vi "ErrorHandling.Gui.vi"(6 "~Shutdown visible (T)":bool=TRUE, 8 "error in (no error)":errorcluster, 10 "~ErrData":T1, 11 "~Show? (T)":bool=TRUE) -> (0 "error out":errorcluster, 2 "~shutdown?":bool)   [LabVIEW 2016]
uses:
  CitTemplate/citTemplate.errData.ctl
  EventLog/EventLog.EventSource.ctl
  ErrorHandling.Gui.Action.ctl
panel:
  out "_loop":i32(ring)=4
  in  "DetailsButton":bool
  out "~ErrorMessage":string
  in  "OKButton":bool
  in  "ShutdownButton":bool
  out "~ErrorSource":string caption="Source"
  out "~ErrorCode":i32 caption="Code"
  out "~ErrorTime":string caption="Time"
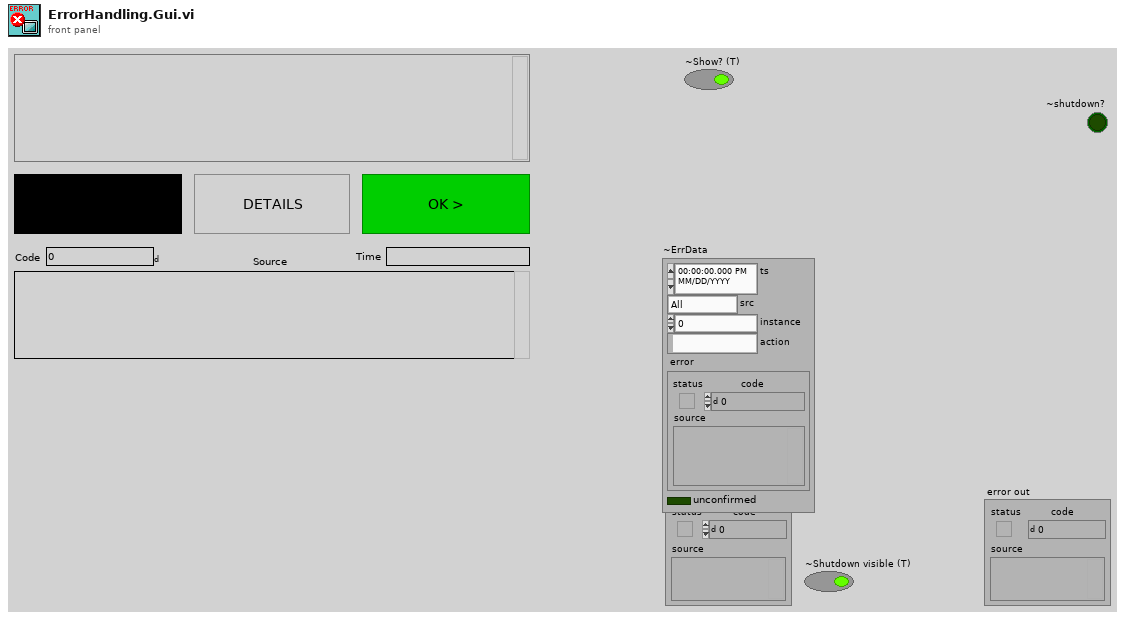
[diagram p1: front panel]
types:
  T1 = typedef "citTemplate.errData.ctl" = cluster{"ts":timestamp, "src":T2, "instance":i32, "action":string, "error":errorcluster, "unconfirmed":bool}
  T2 = typedef "EventLog.EventSource.ctl" = enum16{"All", "Gui", "Cache", "PLC1", "PLC2", "PLC3", "DB", "DB01", "DB02", "DB03", "DB04", "DB05", "DB06", "DB07", "DB08", "DB09", "DB10", "DB11", "DB12", "DB13", "DB14", "DB15", "DB16"}
  T3 = typedef "ErrorHandling.Gui.Action.ctl" = enum32{"idle", "constructor", "destructor", "--- ErrorGUI ---"}
  T4 = enum32{"invalid app kind", "Development System", "Run Time System", "Student Edition", "Embedded LabVIEW", "Evaluation", "Custom"}
  T5 = enum32{"Invalid", "Standard", "Closed", "Hidden", "Minimized", "Maximized"}
  T6 = typedef "LVRectTypeDef.ctl" = cluster{"Left":i16, "Top":i16, "Right":i16, "Bottom":i16}
  T7 = typedef "LVPositionTypeDef.ctl" = cluster{"Left":i32, "Top":i32}
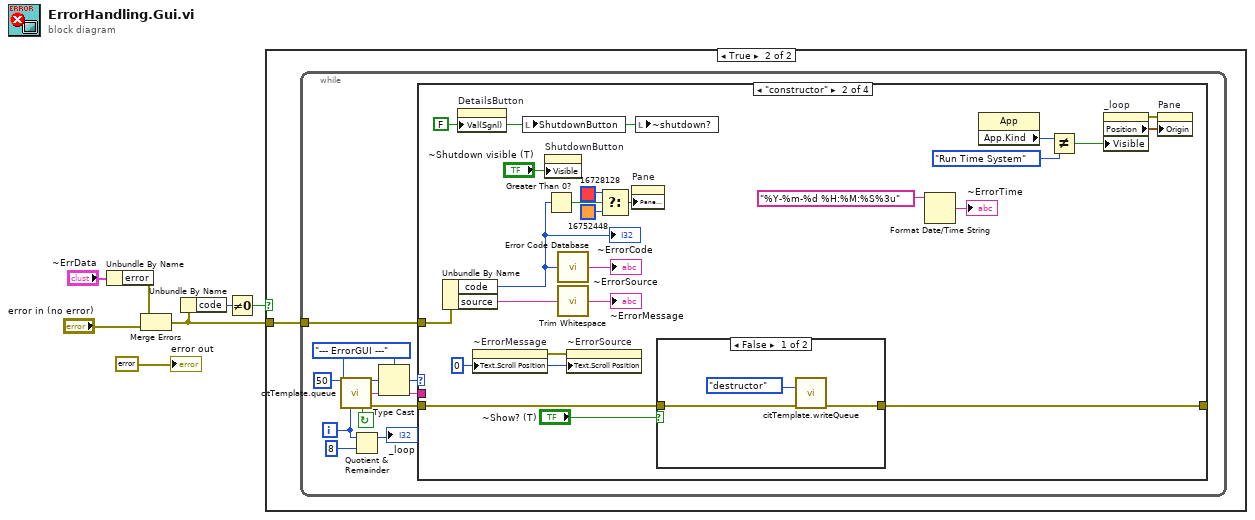
[diagram p0: block diagram]
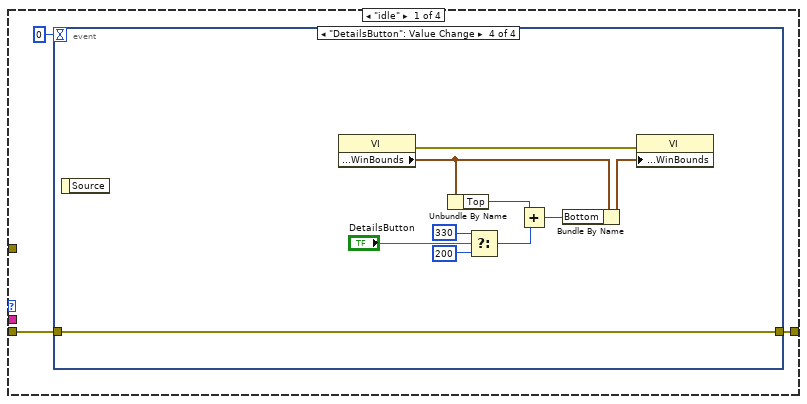
[diagram p3: hidden frame]
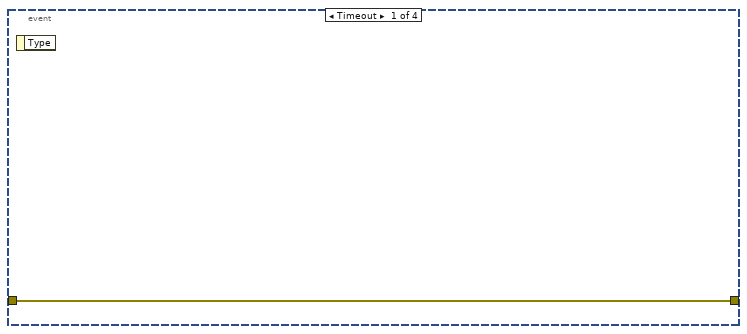
[diagram p4: hidden frame]
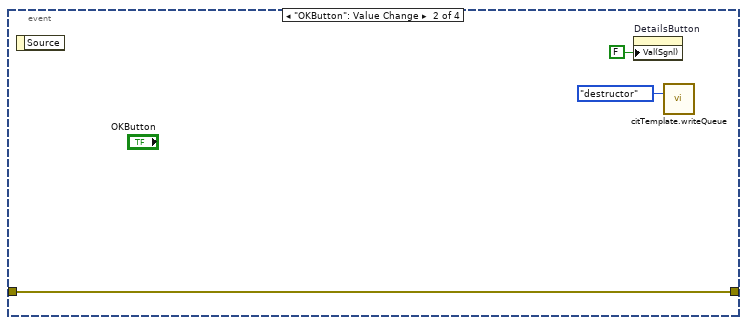
[diagram p5: hidden frame]
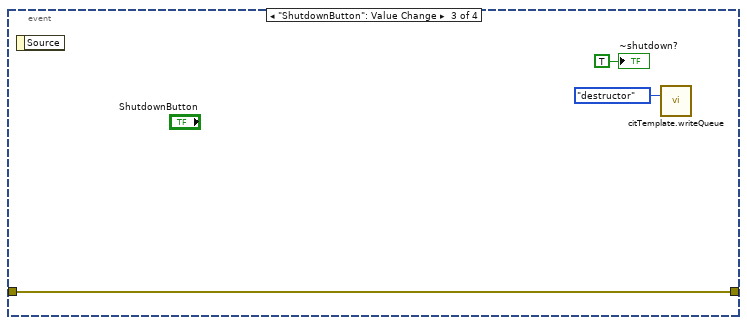
[diagram p6: hidden frame]
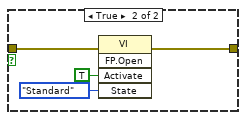
[diagram p7: hidden frame]
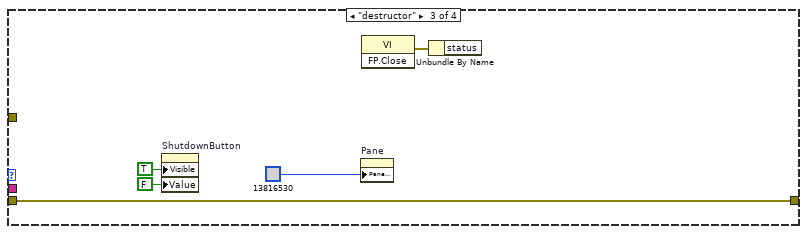
[diagram p8: hidden frame]
diagram:
  n1 = Unbundle By Name("~ErrData") -> ("error"=w2:errorcluster)
  n2 = Merge Errors(w2, "error in (no error)") -> (w3:errorcluster)
  n3 = Unbundle By Name(w3) -> ("code"=w4:i32)
  n4 = Not Equal To 0?(x=w4) -> (x != 0?=w1:bool)
  n5 = case shown="True" w1 {
    tunnel: w3 -> [_ w8]
    frame False {
    }
    frame True {
      n6 = while {
        tunnel: w8 -> [w9]
        i -> [w11]
        stop <- w19 continue-if-true
        w13 = ErrorHandling.Gui.Action."--- ErrorGUI ---" ("Action")
        n7 = call "citTemplate.queue.vi"("ms timeout (250 ms)"=50, "event enum"=w13, "iteration (-1)"=w11) -> ("event out"=w17:u32, "(flatten) data out"=w14:string, "continue"=w19:bool, "error out"=w15:errorcluster)  [unwired: 2 in, 7 out]
        n8 = Quotient & Remainder(x=w11, y=8) -> (x-y*floor(x/y)=→"_loop":i32)  [unwired: 1 out]
        n9 = Type Cast(type=w13, x=w17) -> (*(type *) &x=w16:T3)
        n10 = case shown="\"constructor\"" w16 {
          tunnel: [w20 w40 w74 w75] -> _
          tunnel: w15 -> [w21 w41 w74 w75]
          tunnel: w14 -> [_ _ _ _]
          tunnel: w9 -> [_ w53 _ _]
          frame "idle" {
            n11 = event shown="[3] \"DetailsButton\": Value Change" {
              selector: _ -> [_ _ _ _]
              dyn-events: _ -> [_ _ _ _]
              timeout: 0 -> [_ _ _ _]
              tunnel: w21 -> [w23 w25 w29 w30]
              tunnel: [w23 w25 w29 w30] -> w20
              event Timeout {
                n12 = event-data() -> ()  [unwired: 2 out]
              }
              event "OKButton": Value Change {
                n13 = event-data() -> ()  [unwired: 2 out]
                n14 = property on="DetailsButton" class="Bool (strict)"("Val(Sgnl)"=FALSE ("Value (Signaling)")) -> ()  [unwired: 2 in, 2 out]
                n15 = call "citTemplate.writeQueue.vi"("event in (if not connected:all statemachine with data event)"=ErrorHandling.Gui.Action."destructor" ("Action")) -> ()  [unwired: 4 in, 11 out]
              }
              event "ShutdownButton": Value Change {
                n16 = event-data() -> ()  [unwired: 2 out]
                n17 = call "citTemplate.writeQueue.vi"("event in (if not connected:all statemachine with data event)"=ErrorHandling.Gui.Action."destructor" ("Action")) -> ()  [unwired: 4 in, 11 out]
                "~shutdown?" <- TRUE ("~shutdown?")
              }
              event "DetailsButton": Value Change {
                n18 = event-data() -> ()  [unwired: 2 out]
                n19 = property class="VI"() -> (error out=w37:errorcluster, "Front Panel.WinBounds"=w38:T6)  [unwired: 2 in, 1 out]
                n20 = Unbundle By Name(w38) -> ("Top"=w32:i16)
                n21 = Select(t=i16 330 ("y"), s="DetailsButton", f=i16 200 ("y")) -> (s? t:f=w36:i16)
                n22 = Add(x=w32, y=w36) -> (x+y=w33:i16)
                n23 = Bundle By Name(cluster=w38, "Bottom"=w33) -> (w39:T6)
                n24 = property class="VI"(error in=w37, "Front Panel.WinBounds"=w39) -> ()  [unwired: 1 in, 2 out]
              }
            }
          }
          frame "constructor" {
            w62 = u32 0 ("Text.Scroll Position")
            w46 = FALSE ("Value (Signaling)")
            n25 = Unbundle By Name(w53) -> ("code"=w52:i32, "source"=w50:string)
            "~ErrorCode" <- w52
            n26 = property on="DetailsButton" class="Bool (strict)"("Val(Sgnl)"=w46) -> ()  [unwired: 2 in, 2 out]
            n27 = property on="~ErrorMessage" class="Str"("Text.Scroll Position"=w62) -> (error out=w61:errorcluster)  [unwired: 2 in, 1 out]
            n28 = local write "ShutdownButton"(w46) -> ()
            n29 = property on="ShutdownButton" class="Bool (strict)"("Visible"="~Shutdown visible (T)") -> ()  [unwired: 2 in, 2 out]
            n30 = Greater Than 0?(x=w52) -> (x > 0?=w57:bool)
            n31 = call <vilib>:"Error Code Database.vi"("Error Code"=w52) -> ("Error Text"=→"~ErrorSource":string)
            n32 = call <vilib>:"Trim Whitespace.vi"("string"=w50) -> ("trimmed string"=→"~ErrorMessage":string)  [unwired: 1 in]
            n33 = property on="~ErrorSource" class="Str"(error in=w61, "Text.Scroll Position"=w62) -> ()  [unwired: 1 in, 2 out]
            n34 = Select(t=u32 16728128, s=w57, f=u32 16752448) -> (s? t:f=w56:u32)
            n35 = property on="Pane" class="Pane"("PaneColor"=w56) -> ()  [unwired: 2 in, 2 out]
            n36 = local write "~shutdown?"(w46) -> ()
            n37 = case shown="False" "~Show? (T)" {
              tunnel: w41 -> [w63 w69]
              tunnel: [w65 w68] -> w40
              frame False {
                n38 = call "citTemplate.writeQueue.vi"("event in (if not connected:all statemachine with data event)"=ErrorHandling.Gui.Action."destructor" ("Action"), "error in (no error)"=w63) -> ("error out"=w65:errorcluster)  [unwired: 3 in, 10 out]
              }
              frame True {
                n39 = invoke class="VI" method="FP.Open"(error in=w69, "Activate"=TRUE ("Activate?"), "State"=T5."Standard") -> (error out=w68:errorcluster)  [unwired: 2 in, 4 out]
              }
            }
            n40 = Format Date/Time String(time format string (%c)="%Y-%m-%d %H:%M:%S%3u" ("date/time format")) -> (date/time string=→"~ErrorTime":string)  [unwired: 2 out]
            n41 = property class="App"() -> ("App.Kind"=w44:T4)  [unwired: 2 in, 2 out]
            n42 = Not Equal?(x=w44, y=T4."Run Time System") -> (x != y?=w42:bool)
            n43 = property on="_loop" class="Ring (strict)"("Visible"=w42) -> (error out=w48:errorcluster, "Position"=w47:T7)  [unwired: 2 in, 1 out]
            n44 = property on="Pane" class="Pane"(error in=w48, "Origin"=w47) -> ()  [unwired: 1 in, 2 out]
          }
          frame "destructor" {
            n45 = property on="ShutdownButton" class="Bool (strict)"("Visible"=TRUE, "Value"=FALSE ("ShutdownButton")) -> ()  [unwired: 2 in, 2 out]
            n46 = property on="Pane" class="Pane"("PaneColor"=u32 13816530) -> ()  [unwired: 2 in, 2 out]
            n47 = invoke class="VI" method="FP.Close"() -> (error out=w70:errorcluster)  [unwired: 3 in, 2 out]
            n48 = Unbundle By Name(w70) -> ()  [unwired: 1 out]
          }
          frame "--- ErrorGUI ---" {
          }
        }
      }
    }
  }
  "error out" <- errorcluster {"status"=FALSE, "code"=0, "source"=""} ("error out")
